vi "String - XML 2-Byte Encoding.vi"(0 "Number In (2-Bytes -16bits)":i16 format="%x", 3 "Error In":errorcluster) -> (7 "Output (/ Format)":string, 8 "Output 24bits)":u32=15043232 format="%06x", 10 "Error Out":errorcluster)   [LabVIEW 2013]
panel:
  in  "Use Number In":bool=TRUE
  out "16bits":u32 format="%x"
  in  "String In (2-Byte Width)":string
  out "Swapped Bytes":u32=21152 format="%x"
  out "Output  (24bits) 3":i32=32 format="%024b"
  out "Output  (24bits) 2":i32=2560 format="%024b"
  out "Output  (24bits) 1":i32=327680 format="%024b"
  in  "Octet3 (10ZZ ZZZZ) (24bits)":i32=128 format="%024b"
  in  "Octet2 (10YY YYYY) (24bits)":i32=32768 format="%024b"
  out "Output  (24bits)":i32=15043232 format="%024b"
  in  "Octet1 (1110 XXXX) (24bits)":i32=14680064 format="%024b"
  out "Input (21bits)":u32=21152 format="%021b"
  # "Otherwise, if the code point is less than 10000 (16) output the bitwise inclusive OR of bits 13 through 16 with EO16"
  # "E696 B0"
  # "B065"
  # "E58A A0"
  # "A052"
  # "E59DA1"
  # "6157"
  # "°e RaW"
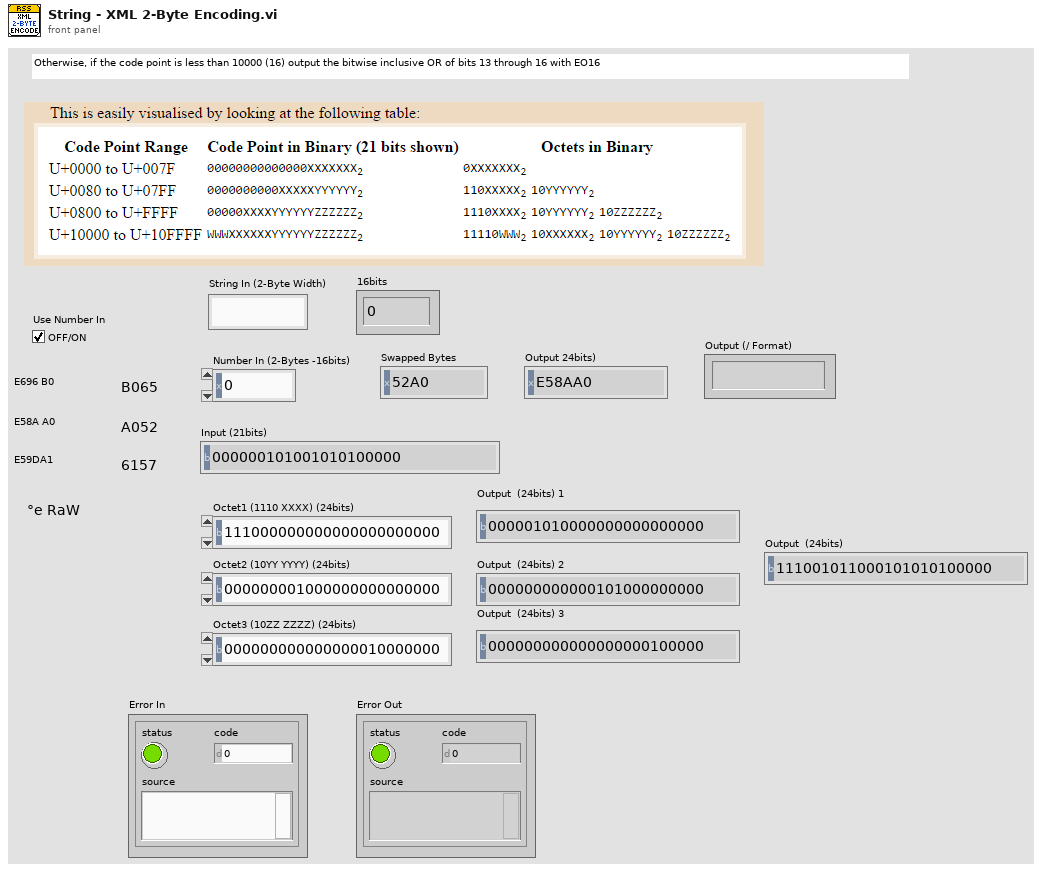
[diagram p1: front panel]
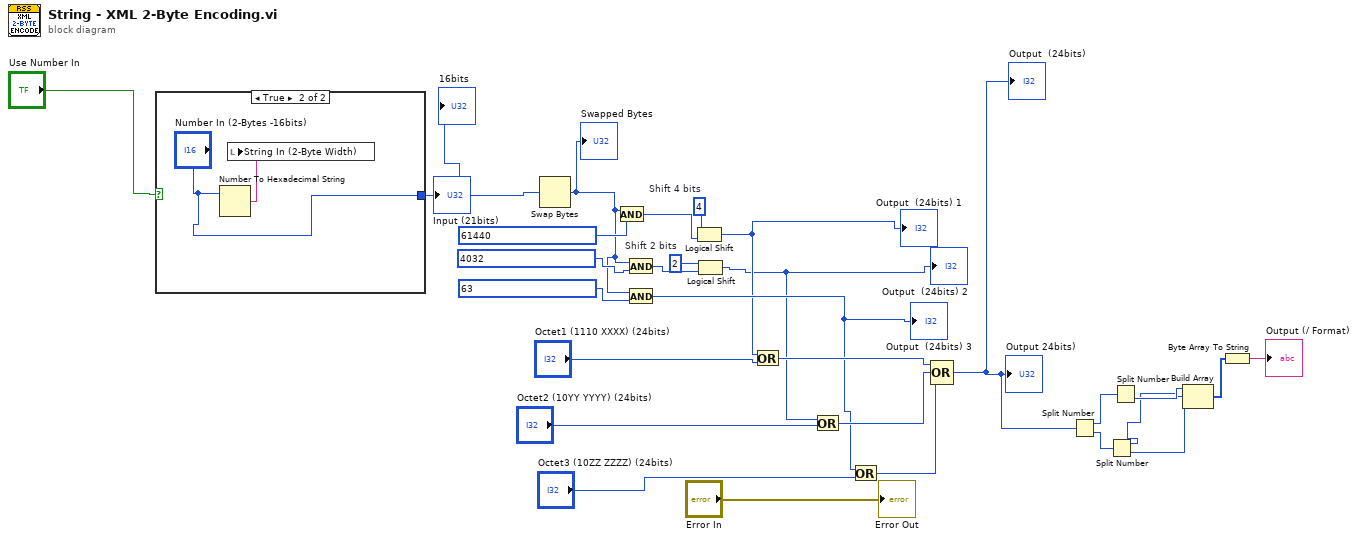
[diagram p0: block diagram]
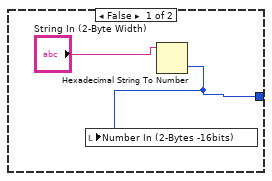
[diagram p2: hidden frame]
diagram:
  w13 = i16 2  # Shift 2 bits
  w17 = i16 4  # Shift 4 bits
  n1 = case shown="True" "Use Number In" {
    tunnel: [w29 "Number In (2-Bytes -16bits)"] -> w10
    frame False {
      n2 = Hexadecimal String To Number(string="String In (2-Byte Width)") -> (number=w29:u32)  [unwired: 2 in, 1 out]
      n3 = local write "Number In (2-Bytes -16bits)"(w29) -> ()
    }
    frame True {
      n4 = Number To Hexadecimal String(2:"Number In (2-Bytes -16bits)") -> (0:w32:string)  [unwired: 1 in]
      n5 = local write "String In (2-Byte Width)"(w32) -> ()
    }
  }
  "Input (21bits)" <- w10
  "16bits" <- w10
  n6 = Swap Bytes(anything=w10) -> (byte swapped=w12:u32)
  "Swapped Bytes" <- w12
  n7 = And(x=w12, y=61440) -> (x .and. y?=w18:u32)
  n8 = And(x=w12, y=i16 4032) -> (x .and. y?=w15:u32)
  n9 = And(x=w12, y=i16 63) -> (x .and. y?=w19:u32)
  "Output  (24bits) 3" <- w19
  n10 = Logical Shift(y=w17, x=w18) -> (x << y=w16:u32)
  "Output  (24bits) 1" <- w16
  n11 = Logical Shift(y=w13, x=w15) -> (x << y=w14:u32)
  "Output  (24bits) 2" <- w14
  n12 = Or(x=w16, y="Octet1 (1110 XXXX) (24bits)") -> (x .or. y?=w22:u32)
  n13 = Or(x=w14, y="Octet2 (10YY YYYY) (24bits)") -> (x .or. y?=w21:u32)
  n14 = Or(x=w19, y="Octet3 (10ZZ ZZZZ) (24bits)") -> (x .or. y?=w20:u32)
  n15 = Compound Arithmetic op=OR(w22, w21, w20) -> (w8:u32)
  "Output  (24bits)" <- w8
  "Output 24bits)" <- w8
  n16 = Split Number(x=w8) -> (hi(x)=w7:u16, lo(x)=w6:u16)
  n17 = Split Number(x=w6) -> (hi(x)=w3:u8, lo(x)=w2:u8)
  n18 = Split Number(x=w7) -> (lo(x)=w4:u8)  [unwired: 1 out]
  n19 = Build Array(w4, w3, w2) -> (w1:u8[])
  n20 = Byte Array To String(unsigned byte array=w1) -> (string=→"Output (/ Format)":string)
  "Error Out" <- "Error In"
